vi "流量计参数设置.vi"(11 "MB session in":refnum<class "MB_Master.lvclass">) -> ()   [LabVIEW 2016, in "流量计集成.lvlib" / "斯坦道功率测流.lvlib"]
uses:
  <vilib>/Plasmionique/MB Master/MB_Master/MB_Master.lvclass
panel:
  in  "写入参数":bool
  in  "读取参数":bool
  in  "关闭":bool
  in  "累积流量清零":bool
  in  "6号机组":bool
  in  "5号机组":bool
  in  "4号机组":bool
  in  "3号机组":bool
  in  "2号机组":bool
  in  "1号机组":bool
  out "水泵效率":dbl
  out "工质密度":dbl
  out "重力加速度":dbl
  out "水泵流量":dbl
  out "水泵扬程":dbl
  out "电机功率":dbl
  in  "Slave ID":u8(ring)=20 items=["1#测流计"=20, "2#测流计"=21]
  # "斯坦道功率测流参数设置"
  # "N=Q.H.g.ρ /η\nN——电机功率，kW\nH——水泵扬程，m\nQ——水泵流量，m^3/s\ng——重力加速度g=9.81\nρ ——工质的密度，当工质是水时，ρ=1\nη——水泵效率，查不到数值时可取η=0.8"
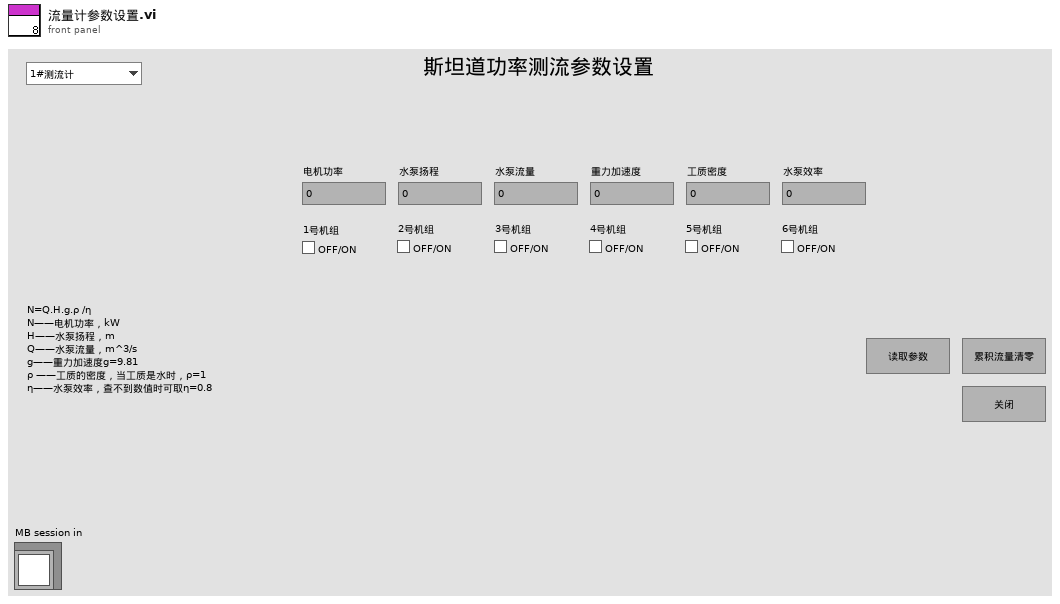
[diagram p1: front panel]
types:
  T1 = typedef "流量计集成.lvlib/斯坦道功率测流.lvlib/测流参数.ctl" = cluster{"电机功率":dbl, "水泵扬程":dbl, "水泵流量":dbl, "重力加速度":dbl, "工质密度":dbl, "水泵效率":dbl, "流量计1启用":u16, "流量计2启用":u16, "流量计3启用":u16, "流量计4启用":u16, "流量计5启用":u16, "流量计6启用":u16, "累积流量清零":u16}
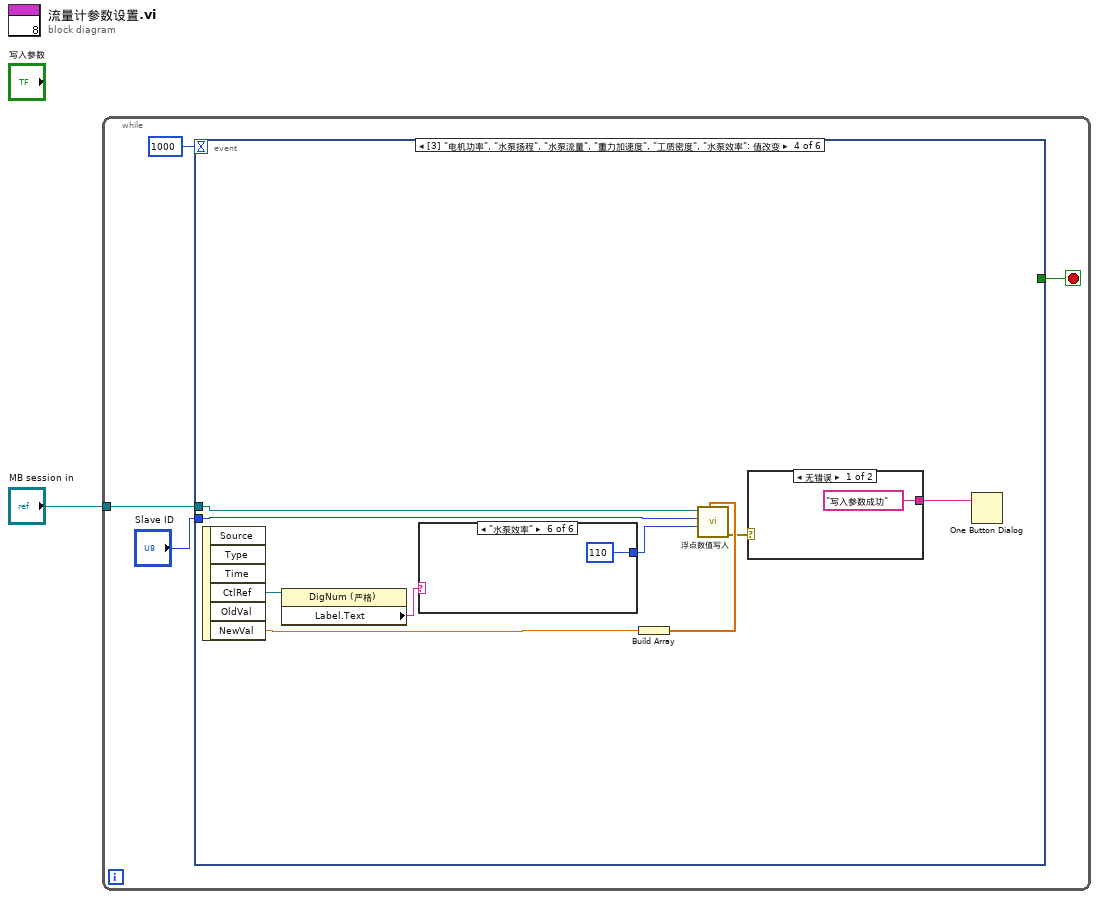
[diagram p0: block diagram]
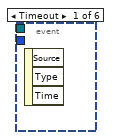
[diagram p2: hidden frame]
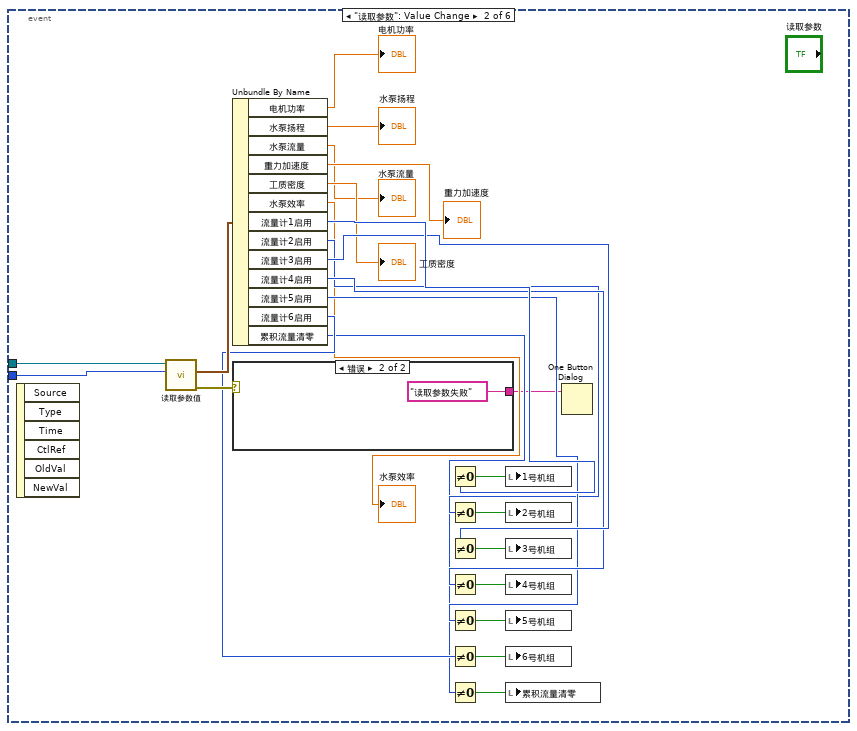
[diagram p3: hidden frame]
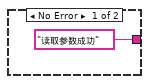
[diagram p4: hidden frame]
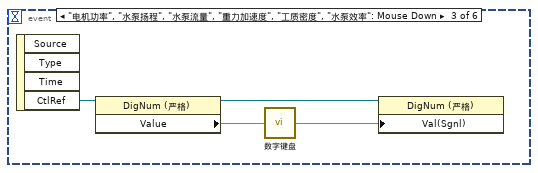
[diagram p5: hidden frame]
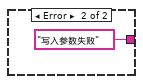
[diagram p6: hidden frame]
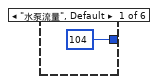
[diagram p7: hidden frame]
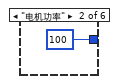
[diagram p8: hidden frame]
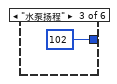
[diagram p9: hidden frame]
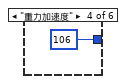
[diagram p10: hidden frame]
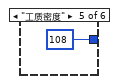
[diagram p11: hidden frame]
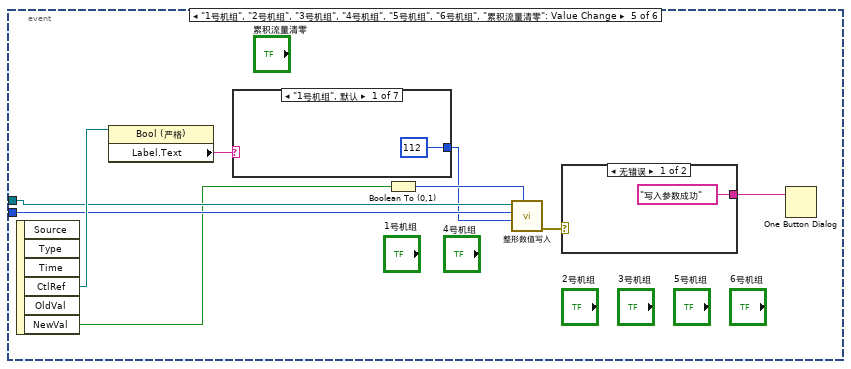
[diagram p12: hidden frame]
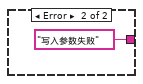
[diagram p13: hidden frame]
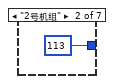
[diagram p14: hidden frame]
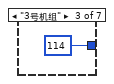
[diagram p15: hidden frame]
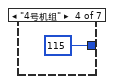
[diagram p16: hidden frame]
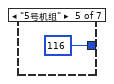
[diagram p17: hidden frame]
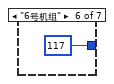
[diagram p18: hidden frame]
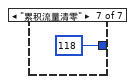
[diagram p19: hidden frame]
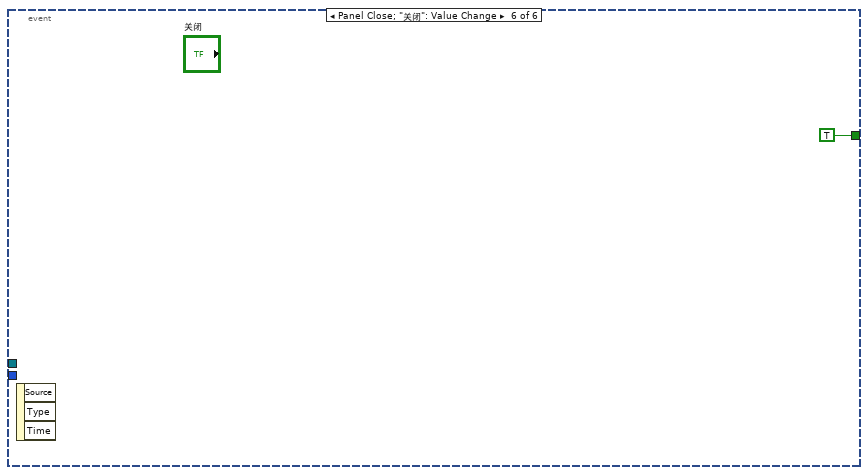
[diagram p20: hidden frame]
diagram:
  n1 = while {
    tunnel: "MB session in" -> [w5]
    stop <- w3 stop-if-true
    n2 = event shown="[3] \"电机功率\", \"水泵扬程\", \"水泵流量\", \"重力加速度\", \"工质密度\", \"水泵效率\": 值改变" {
      selector: _ -> [_ _ _ _ _ _]
      dyn-events: _ -> [_ _ _ _ _ _]
      timeout: 1000 -> [_ _ _ _ _ _]
      tunnel: w5 -> [_ w8 _ w41 w60 _]
      tunnel: [_ _ _ _ _ TRUE] -> w3
      tunnel: "Slave ID" -> [_ w7 _ w45 w59 _]
      event Timeout {
        n3 = event-data() -> ()  [unwired: 1 in, 3 out]
      }
      event "读取参数": Value Change {
        n4 = event-data() -> ()  [unwired: 1 in, 6 out]
        n5 = call "读取参数值.vi"("Slave ID"=w7, "MB session in"=w8) -> ("error out"=w30:errorcluster, "测流参数"=w29:T1)  [unwired: 6 in, 2 out]
        n6 = Unbundle By Name(w29) -> ("电机功率"=→"电机功率":dbl, "水泵扬程"=→"水泵扬程":dbl, "水泵流量"=→"水泵流量":dbl, "重力加速度"=→"重力加速度":dbl, "工质密度"=→"工质密度":dbl, "水泵效率"=→"水泵效率":dbl, "流量计1启用"=w28:u16, "流量计2启用"=w22:u16, "流量计3启用"=w26:u16, "流量计4启用"=w25:u16, "流量计5启用"=w24:u16, "流量计6启用"=w23:u16, "累积流量清零"=w21:u16)
        n7 = case shown="错误" w30 {
          tunnel: ["读取参数成功" ("消息") "读取参数失败" ("消息")] -> w6
          frame No Error {
          }
          frame Error {
          }
        }
        n8 = Not Equal To 0?(x=w28) -> (x != 0?=w27:bool)
        n9 = Not Equal To 0?(x=w22) -> (x != 0?=w20:bool)
        n10 = Not Equal To 0?(x=w26) -> (x != 0?=w19:bool)
        n11 = Not Equal To 0?(x=w25) -> (x != 0?=w18:bool)
        n12 = Not Equal To 0?(x=w24) -> (x != 0?=w17:bool)
        n13 = Not Equal To 0?(x=w23) -> (x != 0?=w16:bool)
        n14 = Not Equal To 0?(x=w21) -> (x != 0?=w15:bool)
        n15 = local write "1号机组"(w27) -> ()
        n16 = local write "2号机组"(w20) -> ()
        n17 = local write "3号机组"(w19) -> ()
        n18 = local write "4号机组"(w18) -> ()
        n19 = local write "5号机组"(w17) -> ()
        n20 = local write "6号机组"(w16) -> ()
        n21 = local write "累积流量清零"(w15) -> ()
        n22 = One Button Dialog(message=w6) -> ()  [unwired: 1 in, 1 out]
      }
      event "电机功率", "水泵扬程", "水泵流量", "重力加速度", "工质密度", "水泵效率": Mouse Down {
        n23 = event-data() -> ("CtlRef"=w36:refnum<vi>)  [unwired: 1 in, 3 out]
        n24 = property class="DigNum (严格)"(reference=w36) -> (reference out=w33:refnum<vi>, "Value"=w35:dbl)  [unwired: 1 in, 1 out]
        n25 = call "数字键盘.vi"("OldNumber"=w35) -> ("NewNumber"=w34:sgl)
        n26 = property class="DigNum (严格)"(reference=w33, "Val(Sgnl)"=w34) -> ()  [unwired: 1 in, 2 out]
      }
      event "电机功率", "水泵扬程", "水泵流量", "重力加速度", "工质密度", "水泵效率": Value Change {
        n27 = event-data() -> ("CtlRef"=w44:refnum<vi>, "NewVal"=w37:dbl)  [unwired: 1 in, 4 out]
        n28 = property class="DigNum (严格)"(reference=w44) -> ("Label.Text"=w43:string)  [unwired: 1 in, 2 out]
        n29 = case shown="\"水泵效率\"" w43 {
          tunnel: [u16 104 ("starting address") u16 100 ("starting address") u16 102 ("starting address") u16 106 ("starting address") u16 108 ("starting address") u16 110 ("starting address")] -> w40
          frame "水泵流量", Default {
          }
          frame "电机功率" {
          }
          frame "水泵扬程" {
          }
          frame "重力加速度" {
          }
          frame "工质密度" {
          }
          frame "水泵效率" {
          }
        }
        n30 = Build Array(w37) -> (w42:dbl[])
        n31 = call "浮点数值写入.vi"("浮点"=w42, "starting address"=w40, "Slave ID"=w45, "MB session in"=w41) -> ("error out"=w38:errorcluster)  [unwired: 6 in, 1 out]
        n32 = case shown="无错误" w38 {
          tunnel: ["写入参数成功" ("消息") "写入参数失败" ("消息")] -> w39
          frame No Error {
          }
          frame Error {
          }
        }
        n33 = One Button Dialog(message=w39) -> ()  [unwired: 1 in, 1 out]
      }
      event "1号机组", "2号机组", "3号机组", "4号机组", "5号机组", "6号机组", "累积流量清零": Value Change {
        n34 = event-data() -> ("CtlRef"=w62:refnum<vi>, "NewVal"=w54:bool)  [unwired: 1 in, 4 out]
        n35 = property class="Bool (严格)"(reference=w62) -> ("Label.Text"=w61:string)  [unwired: 1 in, 2 out]
        n36 = case shown="\"1号机组\", 默认" w61 {
          tunnel: [u16 112 ("starting address") u16 113 ("starting address") u16 114 ("starting address") u16 115 ("starting address") u16 116 ("starting address") u16 117 ("starting address") u16 118 ("starting address")] -> w57
          frame "1号机组", Default {
          }
          frame "2号机组" {
          }
          frame "3号机组" {
          }
          frame "4号机组" {
          }
          frame "5号机组" {
          }
          frame "6号机组" {
          }
          frame "累积流量清零" {
          }
        }
        n37 = Boolean To (0,1)(Boolean=w54) -> (0, 1=w58:i16)
        n38 = call "整形数值写入.vi"("value"=w58, "starting address"=w57, "Slave ID"=w59, "MB session in"=w60) -> ("error out"=w55:errorcluster)  [unwired: 6 in, 1 out]
        n39 = case shown="无错误" w55 {
          tunnel: ["写入参数成功" ("消息") "写入参数失败" ("消息")] -> w56
          frame No Error {
          }
          frame Error {
          }
        }
        n40 = One Button Dialog(message=w56) -> ()  [unwired: 1 in, 1 out]
      }
      event Panel Close; "关闭": Value Change {
        n41 = event-data() -> ()  [unwired: 1 in, 3 out]
      }
    }
  }
